vi "RunningModeTimer.vi"(7 "Initial":bool, 8 "error in (no error)":errorcluster) -> (0 "error out":errorcluster, 2 "TimerOut(s)":dbl)   [LabVIEW 2018]
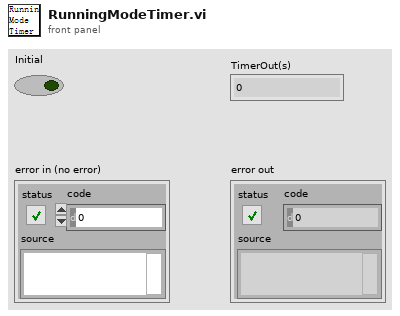
[diagram p1: front panel]
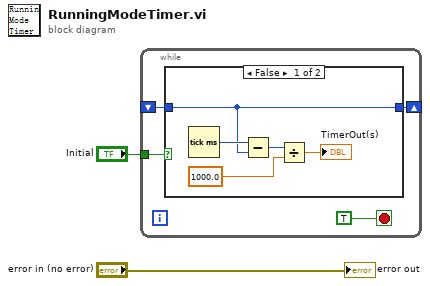
[diagram p0: block diagram]
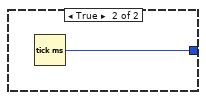
[diagram p2: hidden frame]
diagram:
  n1 = while {
    tunnel: "Initial" -> [w5]
    shift-right: [w4] -> _
    shift-left: _ -> [w3]
    stop <- TRUE stop-if-true
    n2 = case shown="False" w5 {
      tunnel: [w10 w12] -> w4
      tunnel: w3 -> [w10 _]
      frame False {
        n3 = Tick Count (ms)() -> (millisecond timer value=w11:u32)
        n4 = Subtract(x=w11, y=w10) -> (x-y=w9:u32)
        n5 = Divide(x=w9, y=1000.0) -> (x/y=→"TimerOut(s)":dbl)
      }
      frame True {
        n6 = Tick Count (ms)() -> (millisecond timer value=w12:u32)
      }
    }
  }
  "error out" <- "error in (no error)"
